vi "Write Message to Image.vi"(8 "I_Mixed RGB Coordinates":i32[](array[numeric]), 9 "I_Message Bits to Code":u8[](array[numeric]), 10 "I_Message Energy":dbl, 11 "I_Image Data":T1) -> (3 "O_Image Data":T1)   [LabVIEW 2015]
uses:
  <vilib>/picture/picture.llb/imagedata.ctl
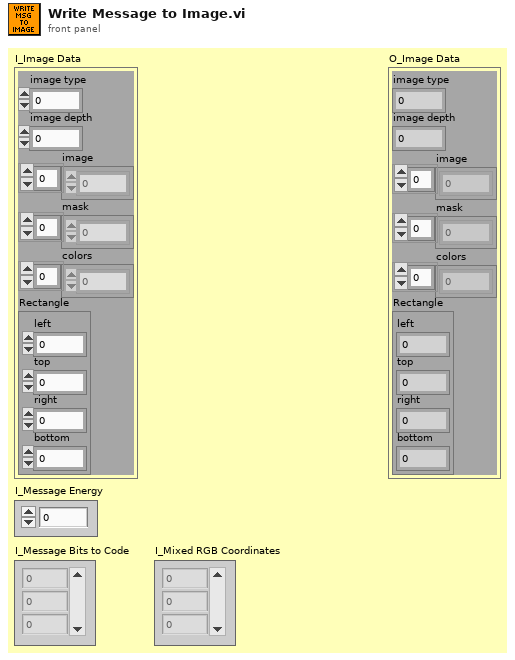
[diagram p1: front panel]
types:
  T1 = typedef "imagedata.ctl" = cluster{"image type":i32, "image depth":i32, "image":u8[], "mask":u8[], "colors":u32[], "Rectangle":cluster{"left":i16, "top":i16, "right":i16, "bottom":i16}}
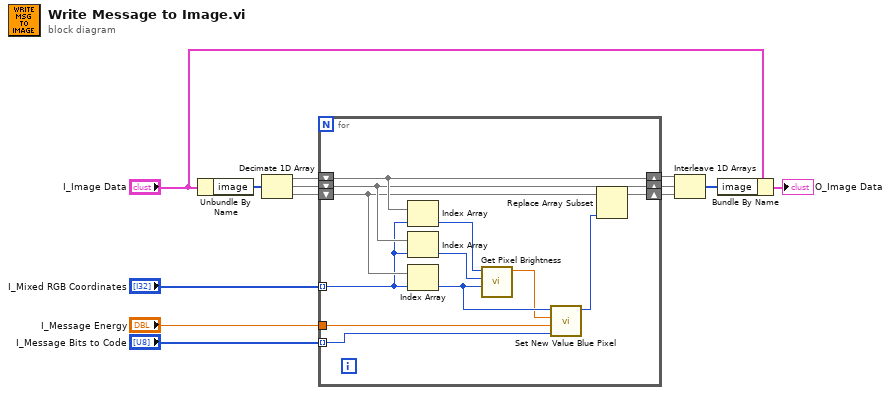
[diagram p0: block diagram]
diagram:
  n1 = Unbundle By Name("I_Image Data") -> ("image"=w13:u8[])
  n2 = Decimate 1D Array(w13) -> (w10:u8[], w11:u8[], w12:u8[])
  n3 = for {
    shift-right: [w24] -> w9
    shift-left: w10 -> [w24]
    shift-right: [w23] -> w8
    shift-left: w11 -> [w23]
    shift-right: [w25] -> w7
    shift-left: w12 -> [w22]
    tunnel: "I_Message Energy" -> [w16]
    tunnel: "I_Message Bits to Code" -> [w15] mode=indexing
    tunnel: "I_Mixed RGB Coordinates" -> [w14] mode=indexing
    n4 = Index Array(array=w24, index=w14) -> (element=w19:u8)
    n5 = Index Array(array=w23, index=w14) -> (element=w20:u8)
    n6 = Index Array(array=w22, index=w14) -> (element=w21:u8)
    n7 = call "Get Pixel Brightness.vi"("B"=w21, "G"=w20, "R"=w19) -> ("Brightness"=w18:dbl)  [unwired: 8 in]
    n8 = call "Set New Value Blue Pixel.vi"("Bit to code"=w15, "Energy"=w16, "General Brightness"=w18, "B"=w21) -> ("New B value Out"=w17:u8)  [unwired: 7 in]
    n9 = Replace Array Subset(array=w22, new element=w17) -> (w25:u8[])  [unwired: 1 in]
  }
  n10 = Interleave 1D Arrays(w9, w8, w7) -> (w6:u8[])
  n11 = Bundle By Name(cluster="I_Image Data", "image"=w6) -> (→"O_Image Data":T1)
